vi "write_clone_kernel.vi"(8 "error in (no error)":errorcluster, 10 "clone_kernel":bool=TRUE, 11 "GaussianProcessClassifier in":refnum<class "GaussianProcessClassifier.lvclass">) -> (0 "error out":errorcluster, 3 "GaussianProcessClassifier out":refnum<class "GaussianProcessClassifier.lvclass">)   [LabVIEW 2020, in "GaussianProcessClassifier.lvclass"]
uses:
  GaussianProcessClassifier.lvclass
  GaussianProcessClassifier.lvclass/GaussianProcessClassifier.ctl
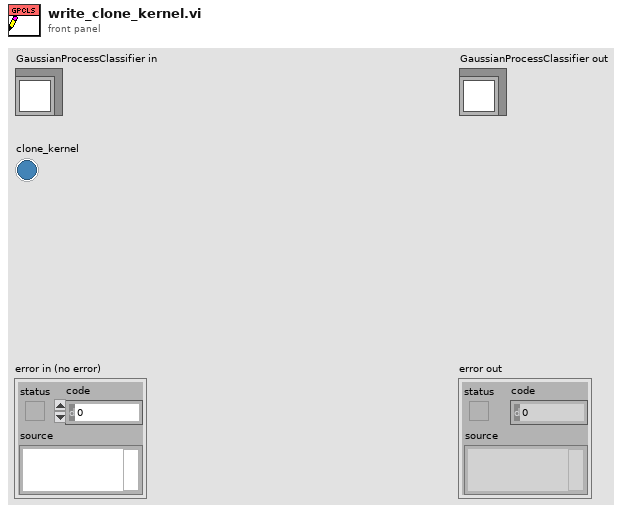
[diagram p1: front panel]
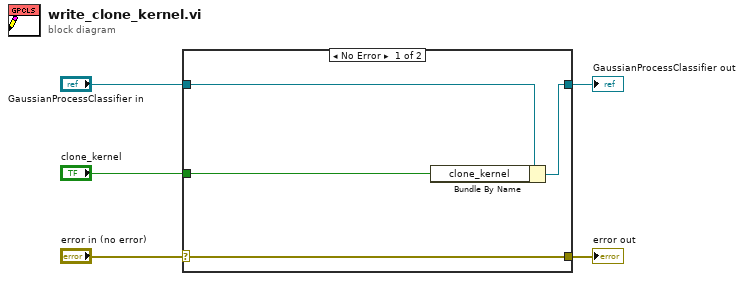
[diagram p0: block diagram]
diagram:
  n1 = case shown="No Error" "error in (no error)" {
    selector: "error in (no error)" -> [w9 w10]
    tunnel: [w9 w10] -> w4
    tunnel: [w7 w11] -> w2
    tunnel: "GaussianProcessClassifier in" -> [w8 w11]
    tunnel: "clone_kernel" -> [w6 _]
    frame No Error {
      n2 = Bundle By Name(cluster=w8, "clone_kernel"=w6) -> (w7:refnum<class "GaussianProcessClassifier.lvclass">)
    }
    frame Error {
    }
  }
  "error out" <- w4
  "GaussianProcessClassifier out" <- w2
